vi "Main On Compile Action VI_Get Buffer Index.vi"(8 "error in":errorcluster, 10 "Channel Ref":T2 format="%.0x", 11 "Device Ref in":T2 format="%.0x") -> (0 "error out":errorcluster, 2 "Channel FIFO Buffer Index":i32, 3 "Device Ref out":T2 format="%.0x", 4 "Found":bool, 5 "FIFO Buffer":T1)   [LabVIEW 2017, in "GE_RM_System Explorer.lvlib"]
uses:
  GE_RM_System Explorer.lvlib
  <vilib>/NI Veristand/Custom Device API/Custom Device Item Ref.ctl
  <vilib>/NI Veristand/Custom Device API/Custom Device Channel Type.ctl
  <vilib>/NI Veristand/Custom Device API/Custom Device API.lvlib
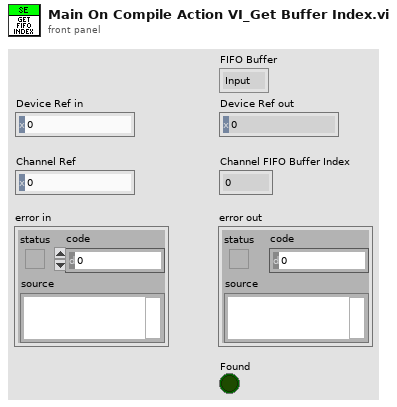
[diagram p1: front panel]
types:
  T1 = typedef "Custom Device API.lvlib/Custom Device Channel Type.ctl" = enum16{"Input", "Output"}
  T2 = typedef "Custom Device API.lvlib/Custom Device Item Ref.ctl" = u64
  T3 = typedef "Custom Device API.lvlib/Custom Device Channel.ctl" = cluster{"Type":T1, "Units":string, "Default Value":dbl, "Faultable":bool, "Scalable":bool}
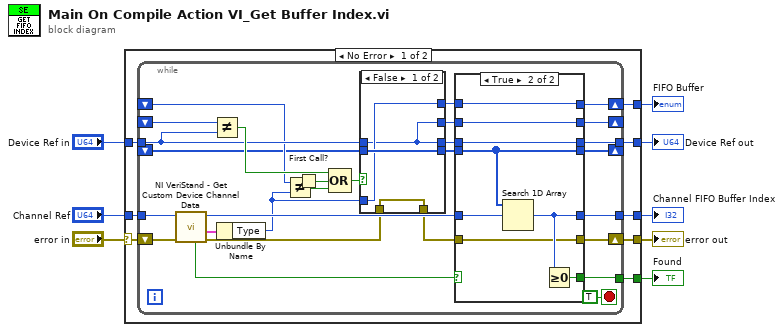
[diagram p0: block diagram]
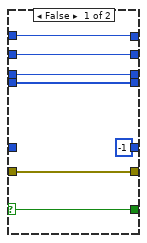
[diagram p2: hidden frame]
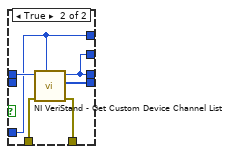
[diagram p3: hidden frame]
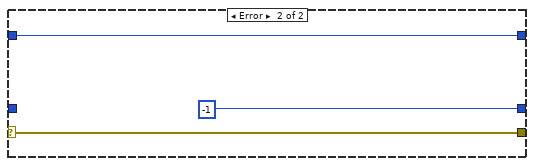
[diagram p4: hidden frame]
diagram:
  n1 = case shown="No Error" "error in" {
    selector: "error in" -> [w11 w70]
    tunnel: [w15 w70] -> w8
    tunnel: [w14 w71] -> w7
    tunnel: [w10 -1 ("index of element")] -> w6
    tunnel: "Channel Ref" -> [w13 _]
    tunnel: [w12 _] -> w4
    tunnel: "Device Ref in" -> [w16 w71]
    tunnel: [w9 _] -> w1
    frame No Error {
      n2 = while {
        tunnel: w13 -> [w41]
        tunnel: [w38] -> w10
        tunnel: [w37] -> w9
        shift-right: [w44] -> w15
        shift-left: w11 -> [w39]
        shift-right: [w22] -> _
        shift-left: _ -> [w34]
        tunnel: w16 -> [w32]
        tunnel: [w43] -> w14
        shift-right: [w28] -> _
        shift-left: _ -> [w20]
        shift-right: [w40] -> w12
        shift-left: _ -> [w21]
        stop <- TRUE stop-if-true
        n3 = call <vilib>:"NI VeriStand - Get Custom Device Channel Data.vi"("error in (no error)"=w39, "Channel Ref in"=w41) -> ("error out"=w18:errorcluster, "Channel"=w31:T3, "Channel Ref out"=w42:T2, "Found"=w36:bool)  [unwired: 6 out]
        n4 = Not Equal?(x=w34, y=w32) -> (x != y?=w33:bool)
        n5 = Unbundle By Name(w31) -> ("Type"=w25:T1)
        n6 = Not Equal?(x=w21, y=w25) -> (x != y?=w26:bool)
        n7 = First Call?() -> (First Call?: T/F=w35:bool)
        n8 = Compound Arithmetic op=OR(w33, w35, w26) -> (w27:bool)
        n9 = case shown="False" w27 {
          tunnel: w32 -> [w61 w69]
          tunnel: [w61 w67] -> w30
          tunnel: [w63 w68] -> w29
          tunnel: w25 -> [w62 w66]
          tunnel: [w62 w66] -> w24
          tunnel: [w61 w67] -> w23
          tunnel: w20 -> [w63 _]
          tunnel: w18 -> [w60 w65]
          tunnel: [w60 w64] -> w17
          frame False {
          }
          frame True {
            n10 = call <vilib>:"NI VeriStand - Get Custom Device Channel List.vi"("Channel Type"=w66, "error in (no error)"=w65, "Device Ref in"=w69) -> ("error out"=w64:errorcluster, "Specified Channel Ref List"=w68:T2[], "Device Ref out"=w67:T2)  [unwired: 6 out]
          }
        }
        n11 = case shown="True" w36 {
          selector: w36 -> [w48 _]
          tunnel: w30 -> [w51 w52]
          tunnel: [w49 w56] -> w44
          tunnel: w17 -> [w49 w56]
          tunnel: [w51 w52] -> w43
          tunnel: w42 -> [_ w59]
          tunnel: [w47 w54] -> w40
          tunnel: [-1 ("index of element") w58] -> w38
          tunnel: [w48 w57] -> w37
          tunnel: w29 -> [w45 w55]
          tunnel: [w45 w55] -> w28
          tunnel: w24 -> [w47 w54]
          tunnel: w23 -> [w46 w53]
          tunnel: [w46 w53] -> w22
          frame False {
          }
          frame True {
            n12 = Search 1D Array(1D array=w55, element=w59) -> (index of element=w58:i32)  [unwired: 1 out]
            n13 = Greater Or Equal To 0?(x=w58) -> (x >= 0?=w57:bool)
          }
        }
      }
    }
    frame Error {
    }
  }
  "Device Ref out" <- w7
  "Channel FIFO Buffer Index" <- w6
  "error out" <- w8
  "FIFO Buffer" <- w4
  "Found" <- w1
